vi "Ev Play Sound.vi"(8 "error in (no error)":errorcluster, 11 "Main Panel in":refnum<class "Main Panel.lvclass">) -> (0 "error out":errorcluster, 3 "Main Panel out":refnum<class "Main Panel.lvclass">)   [LabVIEW 2018, in "Main Panel.lvlib" / "Main Panel.lvclass"]
uses:
  Main Panel.lvclass
  Main Panel.lvclass/Main Panel.ctl
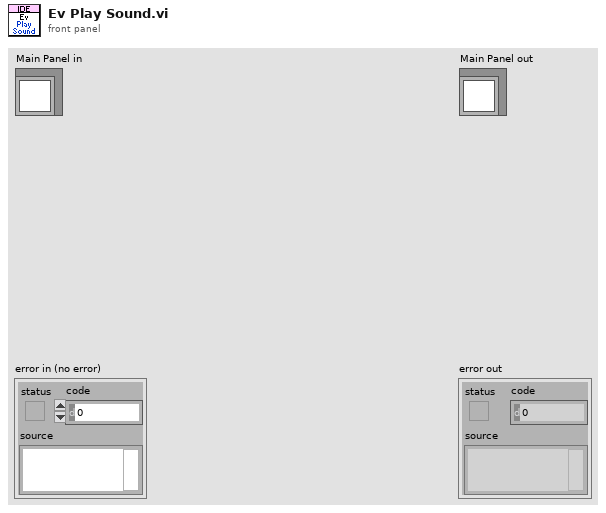
[diagram p1: front panel]
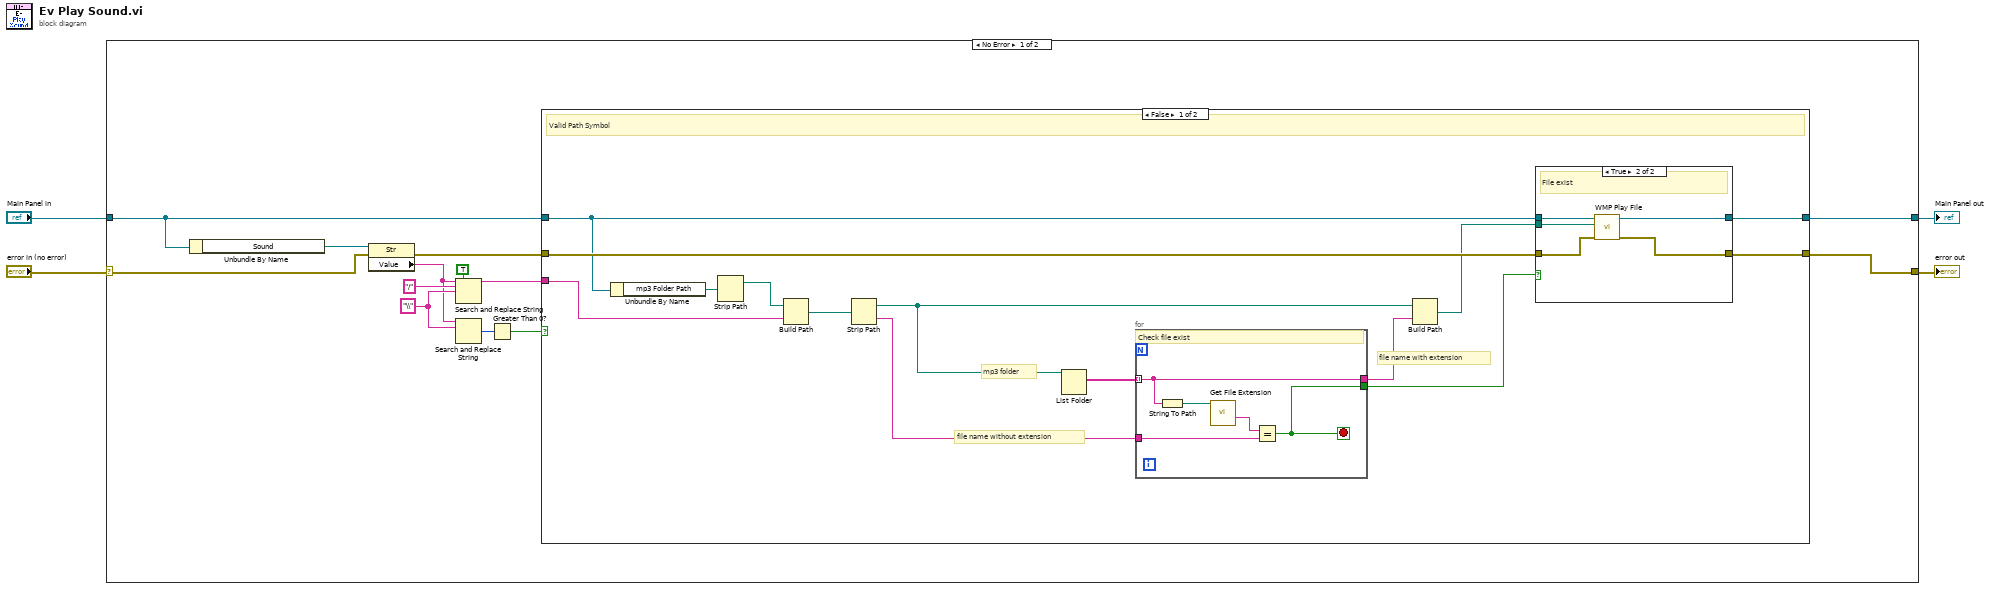
[diagram p0: block diagram]
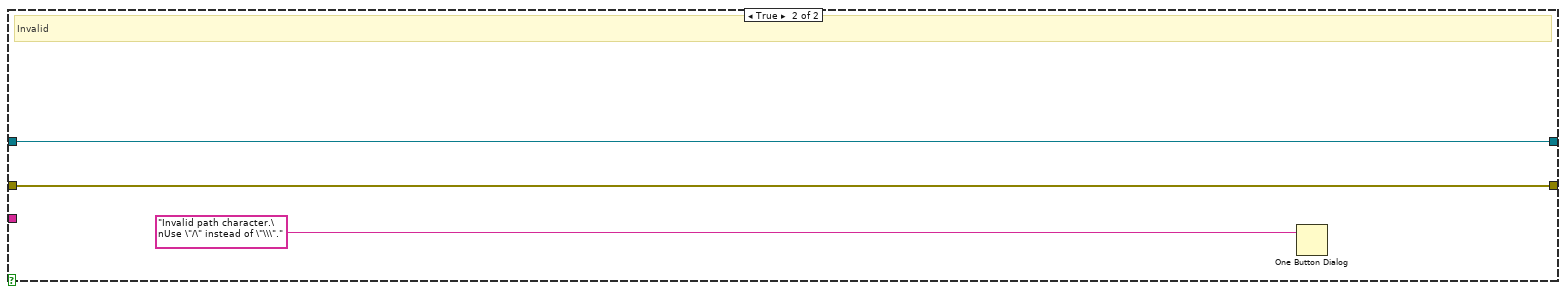
[diagram p3: hidden frame]
diagram:
  n1 = case shown="No Error" "error in (no error)" {
    selector: "error in (no error)" -> [w16 w48]
    tunnel: [w12 w48] -> w3
    tunnel: [w13 w47] -> w1
    tunnel: "Main Panel in" -> [w14 w47]
    frame No Error {
      w8 = "\\" ("search string")
      n2 = Unbundle By Name(w14) -> ("Sound"=w17:refnum<vi>)
      n3 = property class="Str"(reference=w17, error in=w16) -> (error out=w15:errorcluster, "Value"=w5:string)  [unwired: 1 out]
      n4 = Search and Replace String(replace all?=TRUE ("replace all? (F)"), input string=w5, search string="/", replace string=w8) -> (result string=w9:string)  [unwired: 4 in, 3 out]
      n5 = Search and Replace String(input string=w5, search string=w8) -> (number of replacements=w7:i32)  [unwired: 6 in, 3 out]
      n6 = Greater Than 0?(x=w7) -> (x > 0?=w6:bool)
      n7 = case shown="False" w6 {
        tunnel: w15 -> [w31 w45]
        tunnel: w14 -> [w19 w46]
        tunnel: [w30 w46] -> w13
        tunnel: [w29 w45] -> w12
        tunnel: w9 -> [w25 _]
        frame False {
          # "file name with extension"
          # "file name without extension"
          # "mp3 folder"
          # "Valid Path Symbol"
          n8 = Unbundle By Name(w19) -> ("mp3 Folder Path"=w18:path)
          n9 = Strip Path(path=w18) -> (stripped path=w27:path)  [unwired: 1 out]
          n10 = Build Path(base path=w27, name or relative path=w25) -> (appended path=w28:path)
          n11 = Strip Path(path=w28) -> (stripped path=w23:path, name=w24:string)
          n12 = List Folder(path=w23) -> (filenames=w26:string[])  [unwired: 3 in, 3 out]
          n13 = for {
            tunnel: w26 -> [w33] mode=indexing
            tunnel: w24 -> [w35]
            tunnel: [w33] -> w22 if=w32
            tunnel: [w32] -> w21
            stop <- w32 stop-if-true
            # "Check file exist"
            n14 = String To Path(string=w33) -> (path=w36:path)
            n15 = call <vilib>:"Get File Extension.vi"("file"=w36) -> ("filename without extension"=w34:string)  [unwired: 6 in, 4 out]
            n16 = Equal?(x=w34, y=w35) -> (x = y?=w32:bool)
          }
          n17 = Build Path(base path=w23, name or relative path=w22) -> (appended path=w20:path)
          n18 = case shown="True" w21 {
            tunnel: w31 -> [w38 w41]
            tunnel: w19 -> [w37 w43]
            tunnel: [w37 w42] -> w30
            tunnel: [w38 w40] -> w29
            tunnel: w20 -> [_ w39]
            frame False {
              # "Not found"
            }
            frame True {
              # "File exist"
              n19 = call "WMP Play File.vi"("error in (no error)"=w41, "File Path"=w39, "Main Panel in"=w43) -> ("error out"=w40:errorcluster, "Main Panel out"=w42:refnum<class "Main Panel.lvclass">)  [unwired: 7 in]
            }
          }
        }
        frame True {
          # "Invalid"
          n20 = One Button Dialog(message="Invalid path character.\nUse \"/\" instead of \"\\\".") -> ()  [unwired: 1 in, 1 out]
        }
      }
    }
    frame Error {
    }
  }
  "error out" <- w3
  "Main Panel out" <- w1
